vi "Record_MFC_PID_time.vi"(3 "SSH password":string, 4 "Transfer and Run Date Folder After Experiment":bool, 5 "SSH user name":string, 6 "Tags":string, 7 "Frames":i32, 8 "Convert Power to Voltage":bool, 9 "voltages/power":dbl[](array[numeric]), 10 "parameters":string[](array[string]), 11 "parameters headers":string[](array[string])) -> ()   [LabVIEW 2016]
uses:
  <vilib>/Utility/file.llb/Write To Spreadsheet File (DBL).vi
  <vilib>/Utility/file.llb/Write To Spreadsheet File (string).vi
  <vilib>/Utility/file.llb/Read From Spreadsheet File (string).vi
panel:
  out "Waveform Chart":dbl(graph)
  out "Error":string
  out "Save Directory":path
  in  "stop":bool
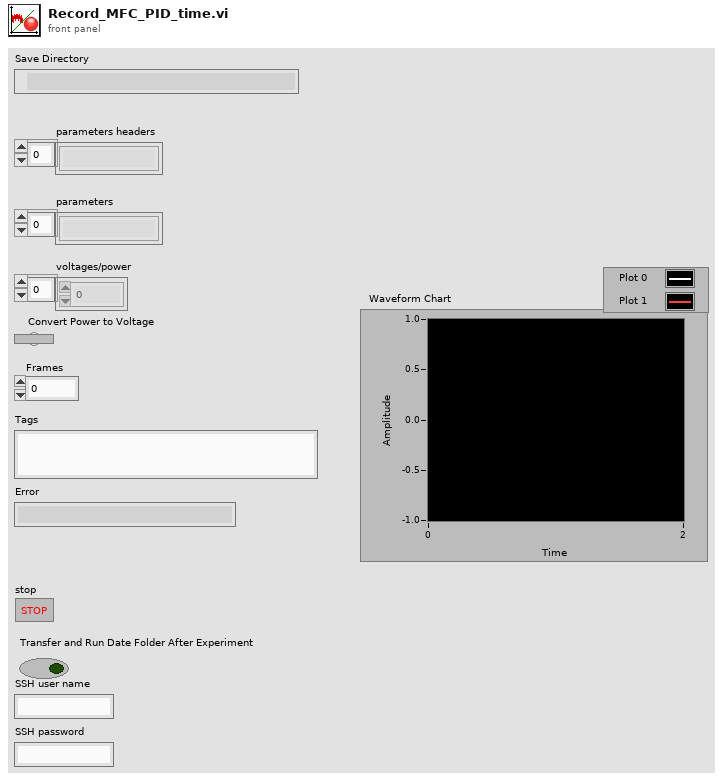
[diagram p1: front panel]
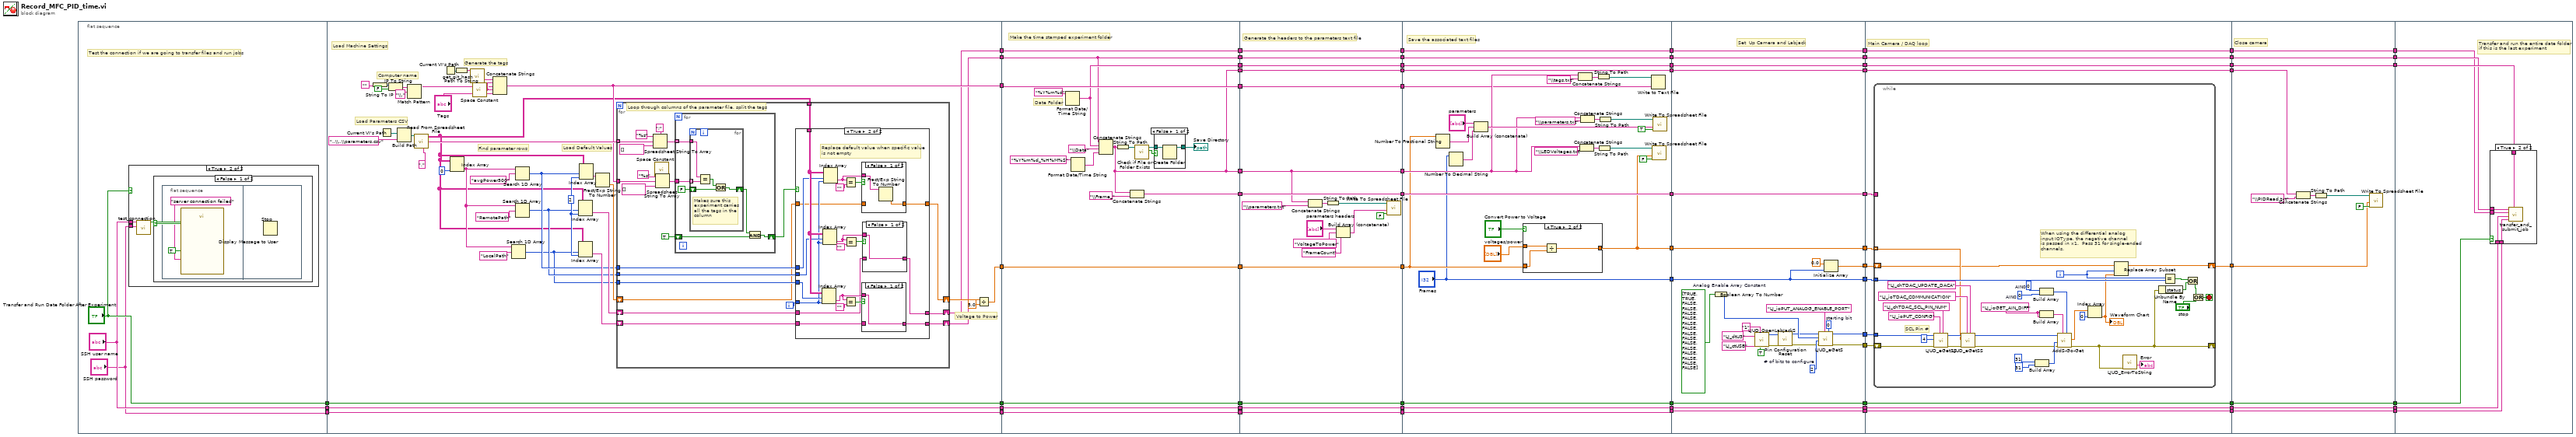
[diagram p0: block diagram]
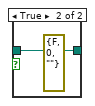
[diagram p8: hidden frame]
diagram:
  n1 = flat-sequence {
    tunnel: ["Transfer and Run Date Folder After Experiment"] -> w31
    tunnel: ["SSH user name"] -> w30
    tunnel: ["SSH password"] -> w29
    tunnel: [w108] -> w61
    tunnel: [w88] -> w60
    tunnel: [w78] -> w51
    tunnel: [w79] -> w50
    tunnel: w31 -> [w99]
    tunnel: w30 -> [w98]
    tunnel: w29 -> [w97]
    tunnel: [w99] -> w22
    tunnel: [w98] -> w15
    tunnel: [w97] -> w14
    tunnel: [w199] -> w45
    tunnel: [w181] -> w43
    tunnel: [w198] -> w41
    tunnel: [w197] -> w39
    tunnel: [w196] -> w37
    tunnel: [w195] -> w35
    tunnel: [w194] -> w33
    tunnel: w50 -> [w194]
    tunnel: w51 -> [w195]
    tunnel: w60 -> [w197]
    tunnel: w61 -> [w198]
    tunnel: [w184] -> w23
    tunnel: w22 -> [w184]
    tunnel: [w183] -> w16
    tunnel: w15 -> [w183]
    tunnel: w14 -> [w182]
    tunnel: [w182] -> w13
    tunnel: [w181] -> w1
    tunnel: w45 -> [w221]
    tunnel: [w221] -> w44
    tunnel: w43 -> [w207]
    tunnel: [w207] -> w42
    tunnel: w41 -> [w220]
    tunnel: [w220] -> w40
    tunnel: w39 -> [w219]
    tunnel: [w219] -> w38
    tunnel: w37 -> [w218]
    tunnel: [w218] -> w36
    tunnel: w35 -> [w217]
    tunnel: [w217] -> w34
    tunnel: w33 -> [w216]
    tunnel: [w216] -> w32
    tunnel: [w206] -> w24
    tunnel: w23 -> [w206]
    tunnel: [w205] -> w17
    tunnel: w16 -> [w205]
    tunnel: w13 -> [w204]
    tunnel: [w204] -> w12
    tunnel: [w203] -> w2
    tunnel: w1 -> [w203]
    tunnel: w44 -> [w249]
    tunnel: [w249] -> w66
    tunnel: [w232] -> w64
    tunnel: ["Frames"] -> w63
    tunnel: w42 -> [w241]
    tunnel: w40 -> [w228]
    tunnel: w38 -> [w223]
    tunnel: w36 -> [w237]
    tunnel: [w237] -> w56
    tunnel: [w236] -> w52
    tunnel: w34 -> [w236]
    tunnel: [w235] -> w46
    tunnel: w32 -> [w235]
    tunnel: [w226] -> w25
    tunnel: w24 -> [w226]
    tunnel: [w225] -> w18
    tunnel: w17 -> [w225]
    tunnel: w12 -> [w224]
    tunnel: [w224] -> w11
    tunnel: [w222] -> w3
    tunnel: w2 -> [w222]
    tunnel: w66 -> [w282]
    tunnel: [w282] -> w69
    tunnel: [w262] -> w68
    tunnel: [w260] -> w67
    tunnel: [w278] -> w65
    tunnel: w64 -> [w278]
    tunnel: w63 -> [w259]
    tunnel: [w259] -> w62
    tunnel: [w274] -> w57
    tunnel: w56 -> [w274]
    tunnel: [w273] -> w53
    tunnel: w52 -> [w273]
    tunnel: [w272] -> w47
    tunnel: w46 -> [w272]
    tunnel: [w271] -> w26
    tunnel: w25 -> [w271]
    tunnel: [w270] -> w19
    tunnel: w18 -> [w270]
    tunnel: w11 -> [w269]
    tunnel: [w269] -> w10
    tunnel: [w258] -> w7
    tunnel: [w257] -> w4
    tunnel: w3 -> [w257]
    tunnel: w69 -> [w296]
    tunnel: w68 -> [w295]
    tunnel: w67 -> [w294]
    tunnel: w65 -> [w293]
    tunnel: w62 -> [w292]
    tunnel: [w291] -> w58
    tunnel: w57 -> [w291]
    tunnel: [w290] -> w54
    tunnel: w53 -> [w290]
    tunnel: [w289] -> w48
    tunnel: w47 -> [w289]
    tunnel: [w288] -> w27
    tunnel: w26 -> [w288]
    tunnel: [w287] -> w20
    tunnel: w19 -> [w287]
    tunnel: w10 -> [w286]
    tunnel: [w286] -> w9
    tunnel: w7 -> [w285]
    tunnel: [w284] -> w6
    tunnel: [w283] -> w5
    tunnel: w4 -> [w283]
    tunnel: [w342] -> w59
    tunnel: w58 -> [w342]
    tunnel: [w341] -> w55
    tunnel: w54 -> [w341]
    tunnel: [w340] -> w49
    tunnel: w48 -> [w340]
    tunnel: [w339] -> w28
    tunnel: w27 -> [w339]
    tunnel: [w338] -> w21
    tunnel: w20 -> [w338]
    tunnel: w9 -> [w337]
    tunnel: [w337] -> w8
    tunnel: w6 -> [w332]
    tunnel: w5 -> [w331]
    tunnel: w59 -> [w348]
    tunnel: w55 -> [w347]
    tunnel: w49 -> [w346]
    tunnel: w28 -> [w345]
    tunnel: w21 -> [w344]
    tunnel: w8 -> [w343]
    frame #0 {
      # "Test the connection if we are going to transfer files and run jobs"
      n2 = case shown="True" "Transfer and Run Date Folder After Experiment" {
        tunnel: "SSH password" -> [_ w75]
        tunnel: "SSH user name" -> [_ w73]
        frame False {
        }
        frame True {
          n3 = call "test_connection.vi"("Username"=w73, "Password"=w75) -> ("Connection Successful"=w74:bool)  [unwired: 7 in]
          n4 = case shown="False" w74 {
            frame False {
              n5 = flat-sequence {
                frame #0 {
                  n6 = call "Display Message to User"("Enable"=TRUE, "Message"="server connection failed") -> ()  [unwired: 8 in, 2 out]
                }
                frame #1 {
                  n7 = Stop() -> ()  [unwired: 1 in]
                }
              }
            }
            frame True {
            }
          }
        }
      }
    }
    frame #1 {
      w90 = 2
      # "Generate the tags"
      # "Find parameter rows"
      # "Load Default Values"
      # "Voltage to Power"
      # "Load Parameters CSV"
      # "Computer name"
      # "Load Machine Settings"
      n8 = String To IP(1:"") -> (0:w116:u32)
      n9 = Current VI's Path() -> (path=w111:path)
      n10 = IP To String(1:FALSE, 2:w116) -> (0:w113:string)
      n11 = Build Path(base path=w111, name or relative path="..\\..\\parameters.csv") -> (appended path=w101:path)
      n12 = Match Pattern(string=w113, regular expression="\\.") -> (before substring=w91:string)  [unwired: 1 in, 3 out]
      n13 = call-poly <vilib>:"Read From Spreadsheet File.vi"("delimiter (\\t)"=",", "file path (dialog if empty)"=w101) -> ("first row"=w89:string[], "all rows"=w81:string[][])  [unwired: 5 in, 3 out]
      n14 = Current VI's Path() -> (path=w94:path)
      n15 = Index Array(array=w81, index (col)=0) -> (element=w102:string[])  [unwired: 1 in]
      n16 = Path To String(path=w94) -> (string=w93:string)
      n17 = call "get_git_hash.vi"("VI folder"=w93) -> ("github hash"=w96:string)  [unwired: 10 in]
      n18 = call <vilib>:"Space Constant.vi"() -> ("String"=w95:string)
      n19 = Concatenate Strings(w96, w95, w91, w95, "Tags") -> (w88:string)
      n20 = Search 1D Array(1D array=w102, element="LocalPath") -> (index of element=w82:i32)  [unwired: 1 in]
      n21 = Search 1D Array(1D array=w102, element="RemotePath") -> (index of element=w83:i32)  [unwired: 1 in]
      n22 = Search 1D Array(1D array=w102, element="avgPower500") -> (index of element=w84:i32)  [unwired: 1 in]
      n23 = Index Array(array=w81, index (row)=w83, index (col)=w90) -> (element=w86:string)
      n24 = Index Array(array=w81, index (row)=w82, index (col)=w90) -> (element=w85:string)
      n25 = Index Array(array=w81, index (row)=w84, index (col)=w90) -> (element=w104:string)
      n26 = Fract/Exp String To Number(string=w104) -> (number=w87:dbl)  [unwired: 3 in, 1 out]
      n27 = for {
        tunnel: w89 -> [w139] mode=indexing
        tunnel: w88 -> [w131]
        tunnel: w84 -> [w126]
        tunnel: w83 -> [w125]
        tunnel: w82 -> [w124]
        tunnel: w81 -> [w129]
        shift-right: [w121] -> w80
        shift-left: w87 -> [w122]
        shift-right: [w118] -> w79
        shift-left: w86 -> [w119]
        shift-right: [w117] -> w78
        shift-left: w85 -> [w120]
        i -> [w123]
        # "Loop through columns of the parameter file, split the tags"
        n28 = Spreadsheet String To Array(delimiter (Tab)=";", format string="%s", spreadsheet string=w139, array type (2D Dbl)=string[] []) -> (array=w135:string[])
        n29 = call <vilib>:"Space Constant.vi"() -> ("String"=w133:string)
        n30 = Spreadsheet String To Array(delimiter (Tab)=w133, format string="%s", spreadsheet string=w131, array type (2D Dbl)=string[] []) -> (array=w130:string[])
        n31 = for {
          tunnel: w135 -> [w175] mode=indexing
          tunnel: w130 -> [w174]
          shift-right: [w172] -> w127
          shift-left: TRUE -> [w170]
          n32 = for {
            tunnel: w175 -> [w180]
            tunnel: w174 -> [w179] mode=indexing
            shift-right: [w176] -> w171
            shift-left: FALSE -> [w177]
            # "Makes sure this\nexperiment carries\nall the tags in the\ncolumn"
            n33 = Equal?(x=w180, y=w179) -> (x = y?=w178:bool)
            n34 = Or(x=w178, y=w177) -> (x .or. y?=w176:bool)
          }
          n35 = And(x=w171, y=w170) -> (x .and. y?=w172:bool)
        }
        n36 = case shown="True" w127 {
          tunnel: w122 -> [w142 w155]
          tunnel: [w142 w154] -> w121
          tunnel: w126 -> [_ w161]
          tunnel: w125 -> [_ w160]
          tunnel: w124 -> [_ w159]
          tunnel: w123 -> [_ w158]
          tunnel: w129 -> [_ w162]
          tunnel: [w141 w144] -> w118
          tunnel: [w140 w146] -> w117
          tunnel: w120 -> [w140 w145]
          tunnel: w119 -> [w141 w143]
          frame False {
          }
          frame True {
            # "Replace default value when specific value\nis not empty"
            n37 = Index Array(array=w162, index (row)=w159, index (col)=w158) -> (element=w147:string)
            n38 = Index Array(array=w162, index (row)=w160, index (col)=w158) -> (element=w150:string)
            n39 = Index Array(array=w162, index (row)=w161, index (col)=w158) -> (element=w153:string)
            n40 = Equal?(x=w153, y="") -> (x = y?=w156:bool)
            n41 = Equal?(x=w147, y="") -> (x = y?=w148:bool)
            n42 = Equal?(x=w150, y="") -> (x = y?=w151:bool)
            n43 = case shown="False" w156 {
              tunnel: w155 -> [_ w169]
              tunnel: [w168 w169] -> w154
              tunnel: w153 -> [w167 _]
              frame False {
                n44 = Fract/Exp String To Number(string=w167) -> (number=w168:dbl)  [unwired: 3 in, 1 out]
              }
              frame True {
              }
            }
            n45 = case shown="False" w148 {
              tunnel: w147 -> [w163 _]
              tunnel: [w163 w164] -> w146
              tunnel: w145 -> [_ w164]
              frame False {
              }
              frame True {
              }
            }
            n46 = case shown="False" w151 {
              tunnel: w150 -> [w165 _]
              tunnel: [w165 w166] -> w144
              tunnel: w143 -> [_ w166]
              frame False {
              }
              frame True {
              }
            }
          }
        }
      }
      n47 = Divide(x=w80, y=5.0) -> (x/y=w108:dbl)
    }
    frame #2 {
      # "Make the time stamped experiment folder"
      # "Date Folder"
      n48 = Format Date/Time String(time format string (%c)="%Y%m%d") -> (date/time string=w196:string)  [unwired: 2 in]
      n49 = Format Date/Time String(time format string (%c)="%Y%m%d_%H%M%S") -> (date/time string=w188:string)  [unwired: 2 in]
      n50 = Concatenate Strings(w195, w196, "\\Data", w188) -> (w181:string)
      n51 = String To Path(string=w181) -> (path=w187:path)
      n52 = Concatenate Strings(w181, "\\Frame_") -> (w199:string)
      n53 = call <vilib>:"Check if File or Folder Exists.vi"("path"=w187) -> ("file or folder exists?"=w192:bool, "dup path"=w191:path)  [unwired: 8 in, 1 out]
      n54 = case shown="False" w192 {
        tunnel: [w200 w202] -> w186
        tunnel: w191 -> [w201 w202]
        frame False {
          n55 = Create Folder(path (use dialog)=w201) -> (created path=w200:path)  [unwired: 2 in, 2 out]
        }
        frame True {
          (unwired) errorcluster {"status"=FALSE, "code"=0, "source"=""} ("error out")
        }
      }
      "Save Directory" <- w186
    }
    frame #3 {
      # "Generate the headers to the parameters text file"
      n56 = Concatenate Strings(w207, "\\parameters.txt") -> (w215:string)
      n57 = String To Path(string=w215) -> (path=w214:path)
      n58 = Build Array (concatenate)("parameters headers", "VoltageToPower", "FrameCount") -> (w211:string[])
      n59 = call-poly <vilib>:"Write To Spreadsheet File.vi"("append to file? (new file:F)"=FALSE, "1D data"=w211, "file path (dialog if empty)"=w214) -> ()  [unwired: 5 in, 1 out]
    }
    frame #4 {
      # "Save the associated text files"
      n60 = Number To Fractional String(number=w228) -> (F-format string=w229:string)  [unwired: 3 in]
      n61 = Number To Decimal String(number="Frames") -> (decimal integer string=w230:string)  [unwired: 1 in]
      n62 = Build Array (concatenate)("parameters", w229, w230) -> (w242:string[])
      n63 = case shown="True" "Convert Power to Voltage" {
        tunnel: "voltages/power" -> [w252 w255]
        tunnel: [w252 w253] -> w232
        tunnel: w228 -> [_ w254]
        frame False {
        }
        frame True {
          n64 = Divide(x=w255, y=w254) -> (x/y=w253:dbl[])
        }
      }
      n65 = Concatenate Strings(w241, "\\tags.txt") -> (w239:string)
      n66 = Concatenate Strings(w241, "\\LEDVoltages.txt") -> (w251:string)
      n67 = Concatenate Strings(w241, "\\parameters.txt") -> (w246:string)
      n68 = String To Path(string=w239) -> (path=w238:path)
      n69 = String To Path(string=w251) -> (path=w250:path)
      n70 = String To Path(string=w246) -> (path=w245:path)
      n71 = Write to Text File(file (use dialog)=w238, text=w223) -> ()  [unwired: 2 in, 3 out]
      n72 = call-poly <vilib>:"Write To Spreadsheet File.vi"("append to file? (new file:F)"=FALSE, "1D data"=w232, "file path (dialog if empty)"=w250) -> ()  [unwired: 5 in, 1 out]
      n73 = call-poly <vilib>:"Write To Spreadsheet File.vi"("append to file? (new file:F)"=TRUE, "1D data"=w242, "file path (dialog if empty)"=w245) -> ()  [unwired: 5 in, 1 out]
    }
    frame #5 {
      w265 = 2  # # of bits to configure
      w267 = 0  # starting bit
      w268 = bool[] [TRUE, TRUE, FALSE, FALSE, FALSE, FALSE, FALSE, FALSE, FALSE, FALSE, FALSE, FALSE, FALSE, FALSE, FALSE, FALSE]  # Analog Enable Array Constant
      # "Set  Up Camera and Labjack"
      n74 = Boolean Array To Number(Boolean array=w268) -> (number=w264:u32)
      n75 = call "LJUD_OpenLabJackS.vi"("FirstFound"=TRUE, "Address"="1" ("DeviceType"), "ConnectionType"="LJ_ctUSB", "DeviceType"="LJ_dtU3") -> ("error out"=w275:errorcluster, "Handle"=w276:i32)  [unwired: 5 in, 1 out]
      n76 = call "Pin Configuration Reset.vi"("error in"=w275, "Handle In"=w276) -> ("error out"=w261:errorcluster, "Handle Out"=w263:i32)  [unwired: 8 in]
      n77 = call "LJUD_eGetS.vi"("Channel"=w267, "IOType"="LJ_ioPUT_ANALOG_ENABLE_PORT", "error in"=w261, "x1"=w265, "Value Write"=w264, "Handle In"=w263) -> ("error out"=w260:errorcluster, "Handle Out"=w262:i32)  [unwired: 3 in, 1 out]
      n78 = Initialize Array(0.0, w259) -> (w258:dbl[])
    }
    frame #6 {
      # "Main Camera / DAQ loop"
      n79 = while {
        tunnel: w296 -> [_]
        tunnel: w295 -> [w316]
        shift-right: [w301] -> _
        shift-left: w294 -> [w315]
        tunnel: w293 -> [w314] mode=indexing
        tunnel: w292 -> [w324]
        shift-right: [w300] -> w284
        shift-left: w285 -> [w299]
        i -> [w298]
        stop <- w330 stop-if-true
        w304 = 0  # AIN0
        w309 = 0  # AIN0
        w310 = "LJ_ioGET_AIN_DIFF" ("IOType")
        # "When using the differential analog\ninput IOType, the negative channel\nis passed in x1.  Pass 31 for single-ended\nchannels."
        # "SCL Pin #"
        n80 = call "LJUD_eGetSS.vi"("Channel"="LJ_chTDAC_SCL_PIN_NUM", "IOType"="LJ_ioPUT_CONFIG", "error in"=w315, "Value Write"=4, "Handle In"=w316) -> ("error out"=w317:errorcluster, "Handle Out"=w320:i32)  [unwired: 4 in, 1 out]
        n81 = call "LJUD_eGetSS.vi"("Channel"="LJ_chTDAC_UPDATE_DACA", "IOType"="LJ_ioTDAC_COMMUNICATION", "error in"=w317, "Value Write"=w314, "Handle In"=w320) -> ("error out"=w302:errorcluster, "Handle Out"=w303:i32)  [unwired: 4 in, 1 out]
        n82 = Build Array(31 ("AIN0"), 31 ("AIN1")) -> (w306:i32[])
        n83 = Build Array(w309, w304) -> (w312:i32[])
        n84 = Build Array(w310, w310) -> (w313:string[])
        n85 = call "AddS-Go-Get.vi"("Channels"=w312, "IOTypes"=w313, "error in"=w302, "x1"=w306, "Handle In"=w303) -> ("error out"=w301:errorcluster, "Values Read"=w305:dbl[])  [unwired: 4 in, 1 out]
        n86 = Index Array(array=w305, index=0 ("Index")) -> (element=w297:dbl)
        "Waveform Chart" <- w297
        n87 = Replace Array Subset(array=w299, new element=w297, index=w298) -> (w300:dbl[])
        n88 = call "LJUD_ErrorToString.vi"("error in"=w301) -> ("String"=→"Error":string)  [unwired: 10 in]
        n89 = Unbundle By Name(w301) -> ("status"=w327:bool)
        n90 = Equal?(x=w298, y=w324) -> (x = y?=w326:bool)
        n91 = Or(x=w326, y=w327) -> (x .or. y?=w325:bool)
        n92 = Or(x=w325, y="stop") -> (x .or. y?=w330:bool)
      }
    }
    frame #7 {
      # "Close camera"
      n93 = Concatenate Strings(w331, "\\PIDRead.txt") -> (w336:string)
      n94 = String To Path(string=w336) -> (path=w335:path)
      n95 = call-poly <vilib>:"Write To Spreadsheet File.vi"("append to file? (new file:F)"=FALSE, "1D data"=w332, "file path (dialog if empty)"=w335) -> ()  [unwired: 5 in, 1 out]
    }
    frame #8 {
      # "Transfer and run the entire date folder\nif this is the last experiment"
      n96 = case shown="True" w345 {
        tunnel: w348 -> [_ w353]
        tunnel: w347 -> [_ w352]
        tunnel: w346 -> [_ w351]
        tunnel: w344 -> [_ w350]
        tunnel: w343 -> [_ w349]
        frame False {
        }
        frame True {
          n97 = call "transfer_and_submit_job.vi"("Date Folder"=w353, "Password"=w349, "Username"=w350, "Remote Data Directory"=w351, "Local Data Directory"=w352) -> ()  [unwired: 7 in]
        }
      }
    }
  }
